vi "Write Visible.vi"(8 "error in (no error)":errorcluster, 10 "Visible":bool, 11 "Shield in":refnum<class "Shield.lvclass">) -> (0 "error out":errorcluster, 3 "Shield out":refnum<class "Shield.lvclass">)   [LabVIEW 2021]
uses:
  Shield.lvclass
  C:/Users/poche/Programs/LabVIEW/Snake Game/GameEl_class/GameEl.lvclass
  C:/Users/poche/Programs/LabVIEW/Snake Game/Shield/Shield.lvclass
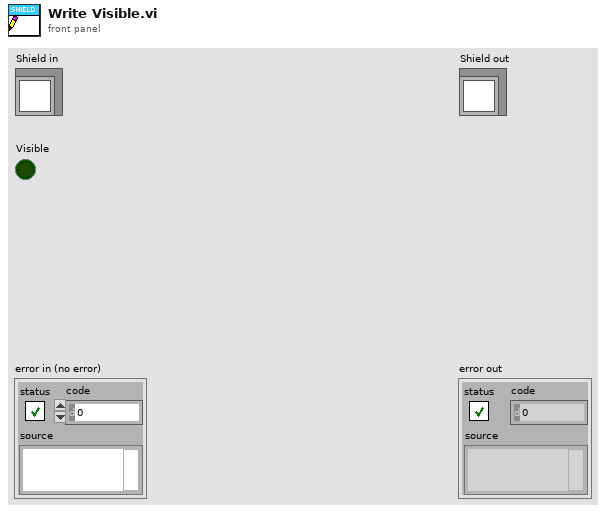
[diagram p1: front panel]
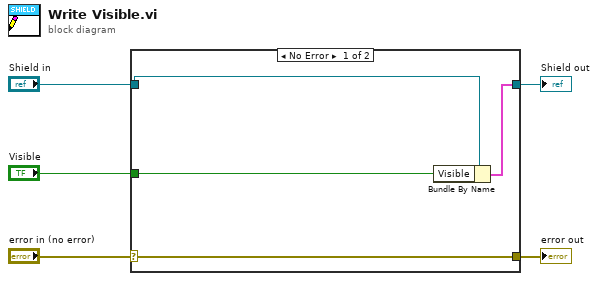
[diagram p0: block diagram]
diagram:
  n1 = case shown="No Error" "error in (no error)" {
    selector: "error in (no error)" -> [w9 w10]
    tunnel: [w9 w10] -> w4
    tunnel: [w7 w11] -> w2
    tunnel: "Shield in" -> [w8 w11]
    tunnel: "Visible" -> [w6 _]
    frame No Error {
      n2 = Bundle By Name(cluster=w8, "Visible"=w6) -> (w7:cluster{})
    }
    frame Error {
    }
  }
  "error out" <- w4
  "Shield out" <- w2
